vi "Silenceable Stateful Dialog.vi"(6 "window title":string="Alert", 7 "config key":string="NI.SilenceDialog", 8 "error in (no error)":errorcluster, 11 "message in":string) -> (0 "error out":errorcluster, 1 "result":T1)   [LabVIEW 2020]
doc: "This VI presents a dialog to the user that allows them to answer a yes-no question or cancel the operation. The dialog includes a \"Do not show this decision again\" checkbox. If user chooses to cancel the operation, this setting is not remembered. If the user answers the question and the checkbox is checked, then the state of the checkbox is remembered in the LabVIEW or built application configuration file along with which button was chosen. In future calls, instead of displaying a dialog, this VI will will return the user's last recorded choice."
uses:
  <vilib>/Silenceable Dialogs/Stateful Dialog Result.ctl
  <resource>/dialog/lvconfig.llb/LV Config Read String.vi
  <resource>/dialog/lvconfig.llb/LV Config Write String.vi
panel:
  in  "error message":string="The config key cannot be an empty string."
  out "message":string
  in  "Do not show this decision again":bool
  in  "No":bool
  in  "Yes":bool
  in  "Cancel":bool
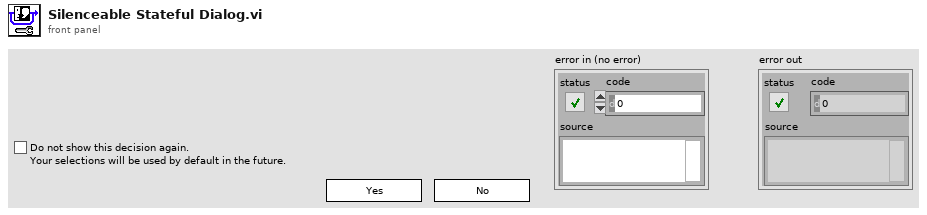
[diagram p1: front panel]
types:
  T1 = typedef "Stateful Dialog Result.ctl" = enum16{"Yes", "No", "Canceled"}
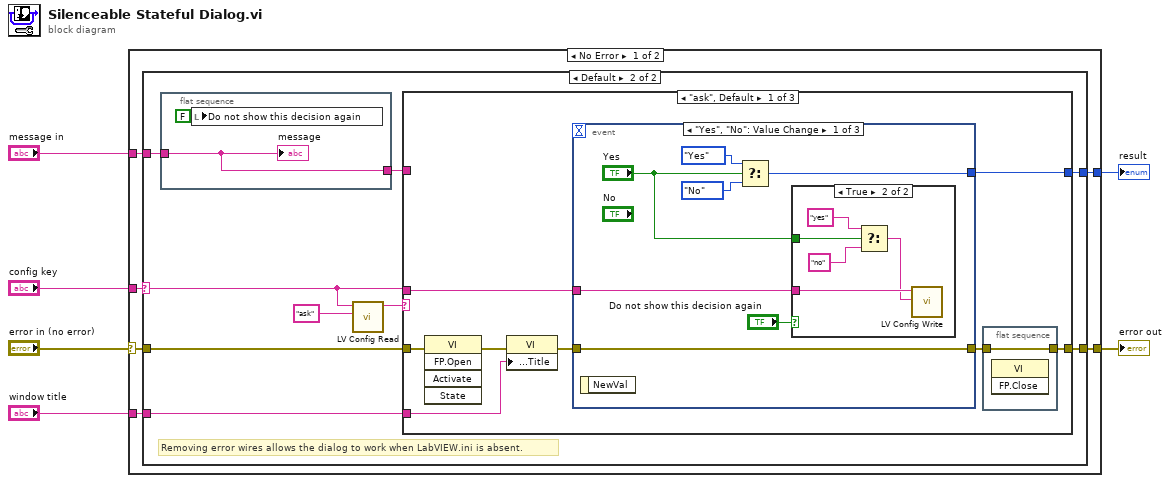
[diagram p0: block diagram]
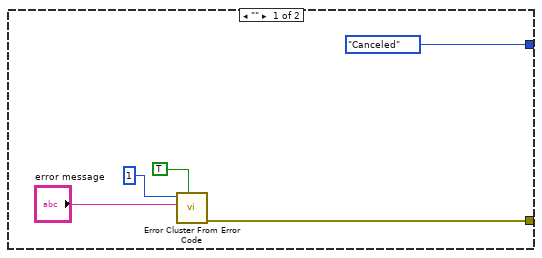
[diagram p2: hidden frame]
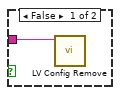
[diagram p3: hidden frame]
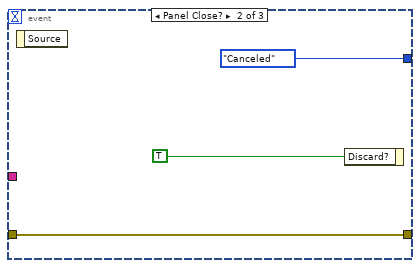
[diagram p4: hidden frame]
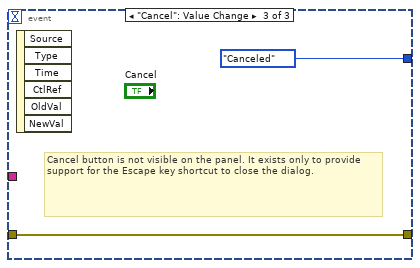
[diagram p5: hidden frame]
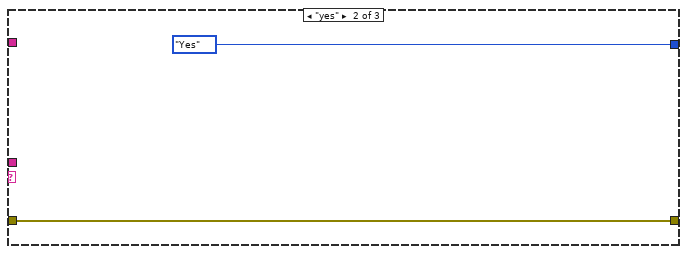
[diagram p6: hidden frame]
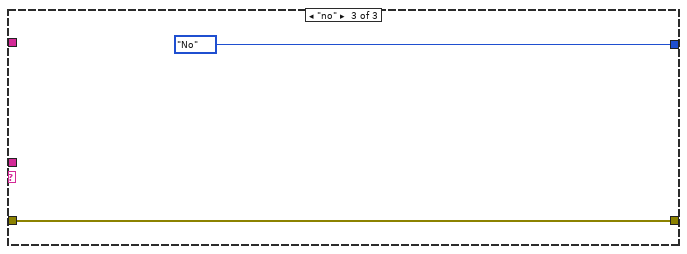
[diagram p7: hidden frame]
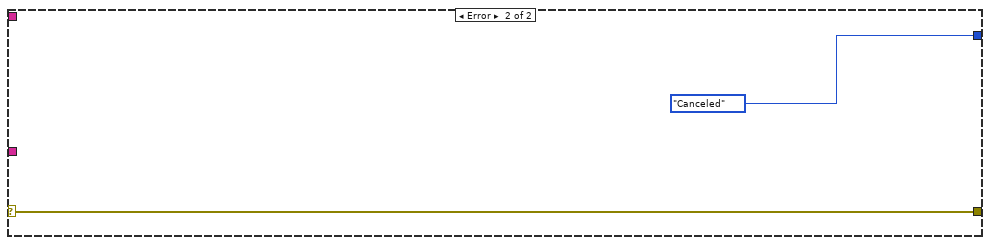
[diagram p8: hidden frame]
diagram:
  n1 = case shown="No Error" "error in (no error)" {
    selector: "error in (no error)" -> [w11 w61]
    tunnel: [w12 w61] -> w5
    tunnel: "config key" -> [w8 _]
    tunnel: "window title" -> [w10 _]
    tunnel: [w9 Stateful_Dialog_Result."Canceled" ("result")] -> w2
    tunnel: "message in" -> [w7 _]
    frame No Error {
      n2 = case shown="Default" w8 {
        selector: w8 -> [_ w20]
        tunnel: [w14 w25] -> w12
        tunnel: w11 -> [_ w24]
        tunnel: w10 -> [_ w22]
        tunnel: [Stateful_Dialog_Result."Canceled" ("result") w21] -> w9
        tunnel: w7 -> [_ w18]
        frame "" {
          n3 = call <vilib>:"Error Cluster From Error Code.vi"("show call chain? (False)"=TRUE, "error message (\"\")"="error message", "error code (0)"=1) -> ("error out"=w14:errorcluster)  [unwired: 6 in]
        }
        frame Default {
          # "Removing error wires allows the dialog to work when LabVIEW.ini is absent."
          n4 = flat-sequence {
            tunnel: [w27] -> w23
            tunnel: w18 -> [w27]
            frame #0 {
              n5 = local write "Do not show this decision again"(FALSE ("Don't show this dialog again.")) -> ()
              "message" <- w27
            }
          }
          n6 = call-poly <resource>:"LV Config Read.vi"("default value"="ask" ("DNL_ask"), "key"=w20) -> ("value"=w26:string)  [unwired: 3 in, 2 out]
          n7 = case shown="\"ask\", Default" w26 {
            tunnel: w20 -> [w36 _ _]
            tunnel: w24 -> [w35 w57 w59]
            tunnel: [w30 w57 w59] -> w25
            tunnel: w23 -> [_ _ _]
            tunnel: w22 -> [w32 _ _]
            tunnel: [w31 Stateful_Dialog_Result."Yes" ("result") Stateful_Dialog_Result."No" ("result")] -> w21
            frame "ask", Default {
              n8 = invoke class="VI" method="FP.Open"(error in=w35) -> (error out=w34:errorcluster)  [unwired: 4 in, 4 out]
              n9 = property class="VI"(error in=w34, "Front Panel.Title"=w32) -> (error out=w33:errorcluster)  [unwired: 1 in, 1 out]
              n10 = event shown="[0] \"Yes\", \"No\": Value Change" {
                selector: _ -> [_ _ _]
                dyn-events: _ -> [_ _ _]
                timeout: _ -> [_ _ _]
                tunnel: w36 -> [w39 _ _]
                tunnel: w33 -> [w43 w52 w55]
                tunnel: [w43 w52 w55] -> w29
                tunnel: [w40 Stateful_Dialog_Result."Canceled" ("result") Stateful_Dialog_Result."Canceled" ("result")] -> w31
                event "Yes", "No": Value Change {
                  n11 = event-data() -> ()  [unwired: 1 in, 1 out]
                  n12 = Select(t=Stateful_Dialog_Result."Yes" ("result"), s="Yes", f=Stateful_Dialog_Result."No" ("result")) -> (s? t:f=w40:T1)
                  n13 = case shown="True" "Do not show this decision again" {
                    tunnel: w39 -> [w45 w50]
                    tunnel: "Yes" -> [_ w46]
                    frame False {
                      n14 = call <resource>:"LV Config Remove.vi"("key"=w45) -> ()  [unwired: 6 in, 1 out]
                    }
                    frame True {
                      n15 = Select(t="yes" ("DNL_yes"), s=w46, f="no" ("DNL_no")) -> (s? t:f=w47:string)
                      n16 = call-poly <resource>:"LV Config Write.vi"("value"=w47, "key"=w50) -> ()  [unwired: 5 in, 1 out]
                    }
                  }
                }
                event Panel Close? {
                  n17 = event-data() -> ()  [unwired: 1 in, 1 out]
                  n18 = event-data("Discard?"=TRUE) -> ()  [unwired: 1 in, 1 out]
                }
                event "Cancel": Value Change {
                  # "Cancel button is not visible on the panel. It exists only to provide support for the Escape key shortcut to close the dialog."
                  n19 = event-data() -> ()  [unwired: 1 in, 6 out]
                }
              }
              n20 = flat-sequence {
                tunnel: [w37] -> w30
                tunnel: w29 -> [w37]
                frame #0 {
                  n21 = invoke class="VI" method="FP.Close"() -> ()  [unwired: 3 in, 3 out]
                }
              }
            }
            frame "yes" {
            }
            frame "no" {
            }
          }
        }
      }
    }
    frame Error {
    }
  }
  "error out" <- w5
  "result" <- w2
